vi "Main.Start.vi"(11 "State Variables in":T1 {"Protocol"."Monitor.Network"."Name" format="%.0x"; "Protocol"."Data"."Trigger.Refs"."Data Reference" format="%.0x"; "Protocol"."Data"."Disable.Refs"."Data Reference" format="%.0x"; "Protocol"."Data"."Timing.Refs"."Data Reference" format="%.0x"; "Protocol"."Data"."Network"."Name" format="%.0x"; "Protocol"."Data"."Incoming.Refs"."Data Reference" format="%.0x"; "Protocol"."Data"."Outgoing.Refs"."Data Reference" format="%.0x"; "Protocol"."XNET.Settings"."Termination" items=["Off", "On"]}) -> (0 "error out":errorcluster, 3 "State Variables out":T1 {"Protocol"."Monitor.Network"."Name" format="%.0x"; "Protocol"."Data"."Trigger.Refs"."Data Reference" format="%.0x"; "Protocol"."Data"."Disable.Refs"."Data Reference" format="%.0x"; "Protocol"."Data"."Timing.Refs"."Data Reference" format="%.0x"; "Protocol"."Data"."Network"."Name" format="%.0x"; "Protocol"."Data"."Incoming.Refs"."Data Reference" format="%.0x"; "Protocol"."Data"."Outgoing.Refs"."Data Reference" format="%.0x"; "Protocol"."XNET.Settings"."Termination" items=["Off", "On"]})   [LabVIEW 2019, in "J1939 Addon Engine.lvlib"]
uses:
  J1939 Addon Engine.lvlib
  Types/Main.State Variables.ctl
  <vilib>/NI/NIVS Inline Async API/_VS Inline Async API/VS Inline Async API/VS Inline Async API.lvclass
  Types/Main.Settings.ctl
  Types/Protocol.App Settings.ctl
  Addon Shared/Types/XNET Settings.ctl
  Addon Shared/Types/Monitor Settings.ctl
  Types/Protocol.XNET Refs.ctl
  <vilib>/NI VeriStand/Custom Device API/Block Data Reference.ctl
  <vilib>/NI VeriStand/Custom Device API/Data Reference.ctl
  Types/Main.Outgoing.Frame.Settings.ctl
  Addon Shared/Types/Outgoing Event Trigger Types.ctl
  SubModules/Frame Protection Support/Source/Shared/Types/Exported Frame Settings.ctl
  SubModules/Frame Protection Support/Source/Shared/Types/Exported Frame Type.ctl
  SubModules/Frame Protection Support/Source/Shared/Types/Exported Protection Settings.ctl
  SubModules/Frame Protection Support/Source/Shared/Types/Protection Type.ctl
  SubModules/Frame Protection Support/Source/Shared/Types/XNET Signal Configuration.ctl
  SubModules/Frame Protection Support/Source/Shared/Types/Exported Counter Settings.ctl
  SubModules/Frame Protection Support/Source/Shared/Types/Exported Event Trigger Type.ctl
  Types/Engine.DTC Settings.ctl
  Addon Shared/Types/Compiled Simulated Settings.ctl
  Types/Engine.DTC FIFOs.ctl
  <vilib>/xnet/xnet.llb/XNET Control Scope.ctl
  <resource>/objmgr/xnet.rc
  <vilib>/NI VeriStand/Custom Device API/Custom Device API.lvlib
  Addon Shared/J1939 Addon Shared.lvlib
  SubModules/Frame Protection Support/Source/Shared/Protection and Counter Support Shared.lvlib
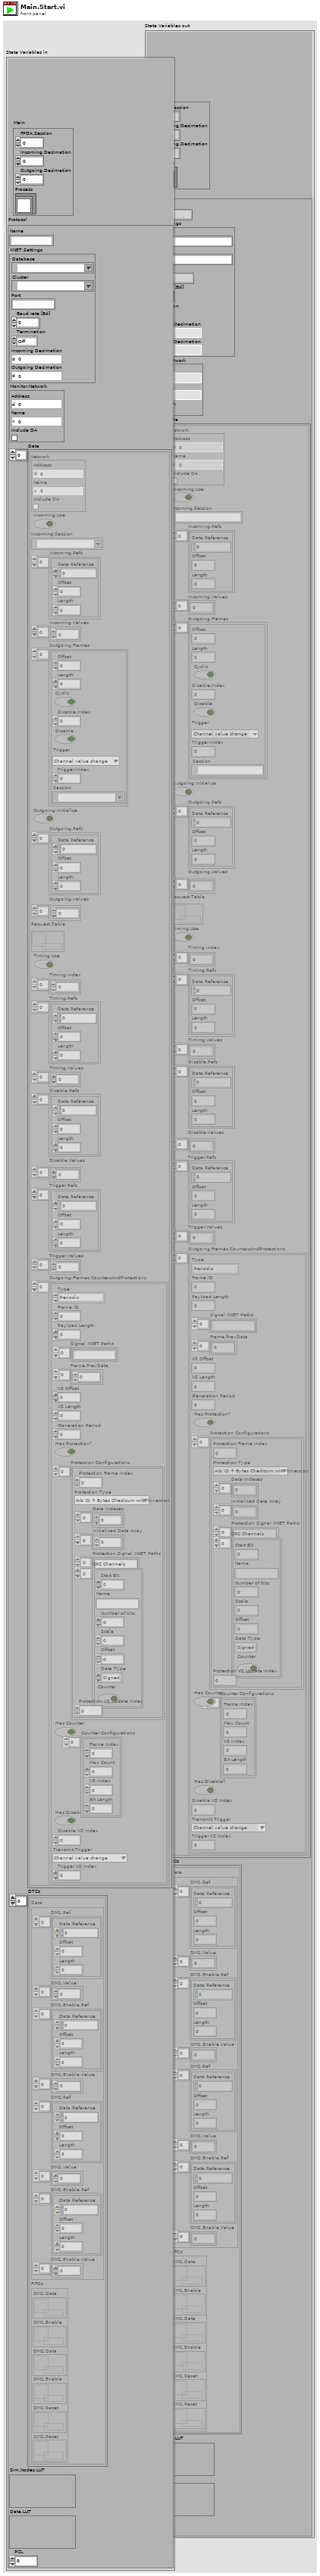
[diagram p1: front panel]
types:
  T1 = typedef "J1939 Addon Engine.lvlib/Main.State Variables.ctl" = cluster{"Main":T2, "Protocol":T3}
  T2 = typedef "J1939 Addon Engine.lvlib/Main.Settings.ctl" = cluster{"FPGA.Session":u32, "Incoming.Decimation":u32, "Outgoing.Decimation":u32, "Process":refnum<class "VS Inline Async API.lvclass">}
  T3 = typedef "J1939 Addon Engine.lvlib/Protocol.App Settings.ctl" = cluster{"Name":string, "XNET.Settings":T4, "Monitor.Network":T5, "Data":T6[], "DTCs":T18[], "Sim.Nodes.LUT":variant, "Data.LUT":variant, "PCL":u32}
  T4 = typedef "J1939 Addon Shared.lvlib/XNET Settings.ctl" = cluster{"Database":refnum<k21>, "Cluster":refnum<k21>, "Port":string, "Baud rate [Bd]":u32, "Termination":u32, "Incoming Decimation":u32, "Outgoing Decimation":u32}
  T5 = typedef "J1939 Addon Shared.lvlib/Monitor Settings.ctl" = cluster{"Address":u8, "Name":u64, "Include DA":bool}
  T6 = typedef "J1939 Addon Engine.lvlib/Protocol.XNET Refs.ctl" = cluster{"Network":T5, "Incoming.Use":bool, "Incoming.Session":refnum<k21>, "Incoming.Refs":T7[], "Incoming.Values":dbl[], "Outgoing.Frames":T9[], "Outgoing.Initialize":bool, "Outgoing.Refs":T7[], "Outgoing.Values":dbl[], "Request.Table":refnum<k33>, "Timing.Use":bool, "Timing.Index":i32[], "Timing.Refs":T7[], "Timing.Values":dbl[], "Disable.Refs":T7[], "Disable.Values":dbl[], "Trigger.Refs":T7[], "Trigger.Values":dbl[], "Outgoing.Frames.CountersAndProtections":T11[]}
  T7 = typedef "Custom Device API.lvlib/Block Data Reference.ctl" = cluster{"Data Reference":T8, "Offset":u64, "Length":u64}
  T8 = typedef "Custom Device API.lvlib/Data Reference.ctl" = i32
  T9 = typedef "J1939 Addon Engine.lvlib/Main.Outgoing.Frame.Settings.ctl" = cluster{"Offset":u32, "Length":u32, "Cyclic":bool, "Disable.Index":i32, "Disable":bool, "Trigger":T10, "Trigger.Index":i32, "Session":refnum<k21>}
  T10 = typedef "J1939 Addon Shared.lvlib/Outgoing Event Trigger Types.ctl" = enum16{"Channel value change", "Trigger channel (not zero)", "Channel value change or trigger channel (not zero)", "Trigger channel (any value change)", "Channel value change or trigger channel (any value change)"}
  T11 = typedef "Protection and Counter Support Shared.lvlib/Exported Frame Settings.ctl" = cluster{"Type":T12, "Frame ID":u32, "Payload Length":u32, "Signal XNET Paths":string[], "Frame.PrevData":dbl[], "VS Offset":i32, "VS Length":i32, "Generation Period":u32, "Has Protection?":bool, "Protection Configurations":T13[], "Has Counter":bool, "Counter Configurations":T16[], "Has Disable?":bool, "Disable VS Index":i32, "Transmit Trigger":T17, "Trigger VS Index":i32}
  T12 = typedef "Protection and Counter Support Shared.lvlib/Exported Frame Type.ctl" = enum16{"Periodic", "Event", "Periodic/Event"}
  T13 = typedef "Protection and Counter Support Shared.lvlib/Exported Protection Settings.ctl" = cluster{"Protection Frame Index":i32, "Protection Type":T14, "Data Indeces":i32[], "Initialized Data Array":dbl[], "Protection Signal XNET Paths":string[], "CRC Channels":T15[], "Protection VS Update Index":i32}
  T14 = typedef "Protection and Counter Support Shared.lvlib/Protection Type.ctl" = enum16{"Arb ID + Bytes Checksum with Inversion", "Arb ID + Bytes CRC with Inversion", "Reversed Raw Signal Checksum with Inversion", "Concatenated Two's Compliment"}
  T15 = typedef "Protection and Counter Support Shared.lvlib/XNET Signal Configuration.ctl" = cluster{"Start Bit":i32, "Name":string, "Number of bits":i32, "Scale":dbl, "Offset":dbl, "Data Type":u32, "Counter":bool}
  T16 = typedef "Protection and Counter Support Shared.lvlib/Exported Counter Settings.ctl" = cluster{"Frame Index":i32, "Max Count":dbl, "VS Index":i32, "Bit Length":i64}
  T17 = typedef "Protection and Counter Support Shared.lvlib/Exported Event Trigger Type.ctl" = enum16{"Channel value change", "Trigger channel (not zero)", "Channel value change or trigger channel (not zero)", "Trigger channel (any value change)", "Channel value change or trigger channel (any value change)"}
  T18 = typedef "J1939 Addon Engine.lvlib/Engine.DTC Settings.ctl" = cluster{"Data":T19, "FIFOs":T20}
  T19 = typedef "J1939 Addon Shared.lvlib/Compiled Simulated Settings.ctl" = cluster{"DM1.Ref":T7[], "DM1.Value":dbl[], "DM1.Enable.Ref":T7[], "DM1.Enable.Value":dbl[], "DM2.Ref":T7[], "DM2.Value":dbl[], "DM2.Enable.Ref":T7[], "DM2.Enable.Value":dbl[]}
  T20 = typedef "J1939 Addon Engine.lvlib/Engine.DTC FIFOs.ctl" = cluster{"DM1.Data":refnum<k33>, "DM1.Enable":refnum<k33>, "DM2.Data":refnum<k33>, "DM2.Enable":refnum<k33>, "DM1.Reset":refnum<k33>, "DM2.Reset":refnum<k33>}
  T21 = typedef "XNET Control Scope.ctl" = u32
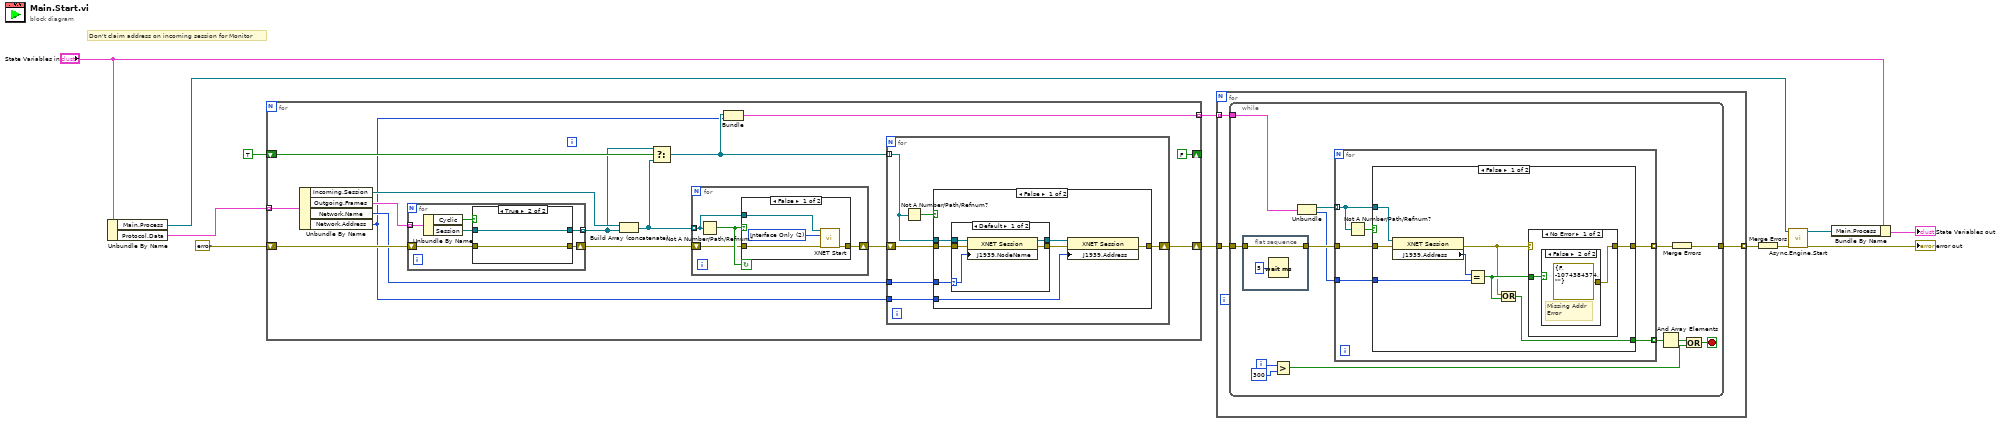
[diagram p0: block diagram]
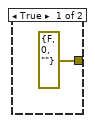
[diagram p2: hidden frame]
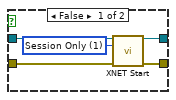
[diagram p8: hidden frame]
diagram:
  # "Don't claim address on incoming session for Monitor"
  n1 = Unbundle By Name("State Variables in") -> ("Main.Process"=w5:refnum<class "VS Inline Async API.lvclass">, "Protocol.Data"=w8:T6[])
  n2 = for {
    shift-right: [w21] -> w10
    shift-left: errorcluster {"status"=FALSE, "code"=0, "source"=""} ("error in (no error)") -> [w26]
    tunnel: w8 -> [w25] mode=indexing
    shift-right: [FALSE] -> _
    shift-left: TRUE -> [w19]
    tunnel: [w13] -> w2 mode=indexing
    n3 = Unbundle By Name(w25) -> ("Incoming.Session"=w24:refnum<k21>, "Outgoing.Frames"=w27:T9[], "Network.Name"=w20:u64, "Network.Address"=w14:u8)
    n4 = for {
      tunnel: w27 -> [w63] mode=indexing
      shift-right: [w61] -> w23
      shift-left: w26 -> [w62]
      tunnel: [w60] -> w18 mode=indexing
      n5 = Unbundle By Name(w63) -> ("Cyclic"=w58:bool, "Session"=w59:refnum<k21>)
      n6 = case shown="True" w58 {
        tunnel: w62 -> [w68 w69]
        tunnel: [w67 w69] -> w61
        tunnel: [w66 w70] -> w60
        tunnel: w59 -> [w65 w70]
        frame False {
          w64 = T21 1 items=["Normal", "Session Only", "Interface Only", "Session Only Blocking"] ("scope (normal)")
          n7 = call <vilib>:"XNET Start.vi"("session in"=w65, "scope (normal)"=w64, "error in (no error)"=w68) -> ("session out"=w66:refnum<k21>, "error out"=w67:errorcluster)  [unwired: 11 in]
        }
        frame True {
        }
      }
    }
    n8 = Build Array (concatenate)(w24, w18) -> (w17:refnum<k21>[])
    n9 = Select(t=w18, s=w19, f=w17) -> (s? t:f=w15:refnum<k21>[])
    n10 = for {
      tunnel: w17 -> [w50] mode=indexing
      shift-right: [w49] -> w22
      shift-left: w23 -> [w51]
      stop <- w52 continue-if-true
      n11 = Not A Number/Path/Refnum?(number/path/refnum=w50) -> (NaN/Path/Refnum?=w52:bool)
      n12 = case shown="False" w52 {
        tunnel: w51 -> [w54 w57]
        tunnel: w50 -> [w55 _]
        tunnel: [w53 w57] -> w49
        frame False {
          w56 = T21 2 items=["Normal", "Session Only", "Interface Only", "Session Only Blocking"] ("scope (normal)")
          n13 = call <vilib>:"XNET Start.vi"("session in"=w55, "scope (normal)"=w56, "error in (no error)"=w54) -> ("error out"=w53:errorcluster)  [unwired: 11 in, 1 out]
        }
        frame True {
        }
      }
    }
    n14 = Bundle(w15, "Address"=w14) -> (w13:cluster{refnum<k21>[], "Address":u8})  [unwired: 1 in]
    n15 = for {
      tunnel: w15 -> [w31] mode=indexing
      shift-right: [w30] -> w21
      shift-left: w22 -> [w32]
      tunnel: w20 -> [w29]
      tunnel: w14 -> [w28]
      n16 = Not A Number/Path/Refnum?(number/path/refnum=w31) -> (NaN/Path/Refnum?=w33:bool)
      n17 = case shown="False" w33 {
        tunnel: w32 -> [w39 w48]
        tunnel: w31 -> [w40 _]
        tunnel: [w38 w48] -> w30
        tunnel: w29 -> [w35 _]
        tunnel: w28 -> [w36 _]
        frame False {
          n18 = case shown="Default" w35 {
            selector: w35 -> [w43 _]
            tunnel: w40 -> [w45 w46]
            tunnel: w39 -> [w44 w47]
            tunnel: [w42 w47] -> w37
            tunnel: [w41 w46] -> w34
            frame Default {
              n19 = property class="XNET Session"(reference=w45, error in=w44, "J1939.NodeName"=w43) -> (reference out=w41:refnum<k21>, error out=w42:errorcluster)
            }
            frame 0 {
            }
          }
          n20 = property class="XNET Session"(reference=w34, error in=w37, "J1939.Address"=w36) -> (error out=w38:errorcluster)  [unwired: 1 out]
        }
        frame True {
        }
      }
    }
  }
  n21 = for {
    tunnel: w10 -> [w73]
    tunnel: [w72] -> w9 mode=indexing
    tunnel: w2 -> [w71] mode=indexing
    n22 = while {
      tunnel: w73 -> [w83]
      tunnel: [w85] -> w72
      tunnel: w71 -> [w76]
      i -> [w81]
      stop <- w77 stop-if-true
      n23 = flat-sequence {
        tunnel: [w88] -> w84
        tunnel: w83 -> [w88]
        frame #0 {
          n24 = Wait (ms)(milliseconds to wait=u32 5) -> ()  [unwired: 1 out]
        }
      }
      n25 = Greater?(x=w81, y=300) -> (0:w78:bool)
      n26 = Unbundle(w76) -> (w74:refnum<k21>[], "Address"=w75:u8)
      n27 = for {
        tunnel: w84 -> [w94]
        tunnel: [w93] -> w86 mode=indexing
        tunnel: w74 -> [w92] mode=indexing
        tunnel: w75 -> [w90]
        tunnel: [w89] -> w80 mode=indexing
        n28 = Not A Number/Path/Refnum?(number/path/refnum=w92) -> (NaN/Path/Refnum?=w91:bool)
        n29 = case shown="False" w91 {
          selector: w91 -> [_ w108]
          tunnel: w94 -> [w100 w109]
          tunnel: [w99 w109] -> w93
          tunnel: w92 -> [w97 _]
          tunnel: w90 -> [w98 _]
          tunnel: [w95 w108] -> w89
          frame False {
            n30 = property class="XNET Session"(reference=w97, error in=w100) -> (error out=w101:errorcluster, "J1939.Address"=w96:u8)  [unwired: 1 out]
            n31 = Equal?(x=w96, y=w98) -> (x = y?=w102:bool)
            n32 = Compound Arithmetic op=OR(w101, w102) -> (w95:bool)
            n33 = case shown="No Error" w101 {
              selector: w101 -> [_ w107]
              tunnel: w102 -> [w104 _]
              tunnel: [w103 w107] -> w99
              frame No Error {
                n34 = case shown="False" w104 {
                  tunnel: [errorcluster {"status"=FALSE, "code"=0, "source"=""} ("error out") errorcluster {"status"=FALSE, "code"=-1074384374, "source"=""} ("error out")] -> w103
                  frame True {
                  }
                  frame False {
                    # "Missing Addr\nError"
                  }
                }
              }
              frame Error {
              }
            }
          }
          frame True {
          }
        }
      }
      n35 = And Array Elements(Boolean array=w80) -> (logical AND=w79:bool)
      n36 = Merge Errors(w86) -> (w85:errorcluster)
      n37 = Compound Arithmetic op=OR(w79, w78) -> (w77:bool)
    }
  }
  n38 = Merge Errors(w9) -> (w7:errorcluster)
  n39 = call <vilib>:"Async.Engine.Start.vi"("error in (no error)"=w7, "VS Inline Async API in"=w5) -> ("error out"=→"error out":errorcluster, "VS Inline Async API out"=w4:refnum<class "VS Inline Async API.lvclass">)  [unwired: 8 in]
  n40 = Bundle By Name(cluster="State Variables in", "Main.Process"=w4) -> (→"State Variables out":T1)
